vi "Joystick interpolation Full.vi"(8 "array":dbl[](array[numeric]), 9 "Numeric":dbl=1000.0 format="%#_13g", 10 "Joystick Sim":dbl(slide) scale=-1.0..1.0, 11 "method":i32(ring)=3 items=["nearest", "linear", "spline", "cubic Hermite", "Lagrange"]) -> (3 "Power":dbl(slide) scale=-1.0..1.0)   [LabVIEW 2017]
uses:
  <vilib>/Analysis/1siggen.llb/Ramp Pattern by Delta.vi
  <vilib>/gmath/NI_Gmath.lvlib
  <vilib>/Analysis/NI_AALBase.lvlib
panel:
  out "Interpolated Data":dbl[][](array[numeric])
  out "1D Interpolation Graph":cluster{"yi":dbl[], "ramp data":dbl[]}[](graph)
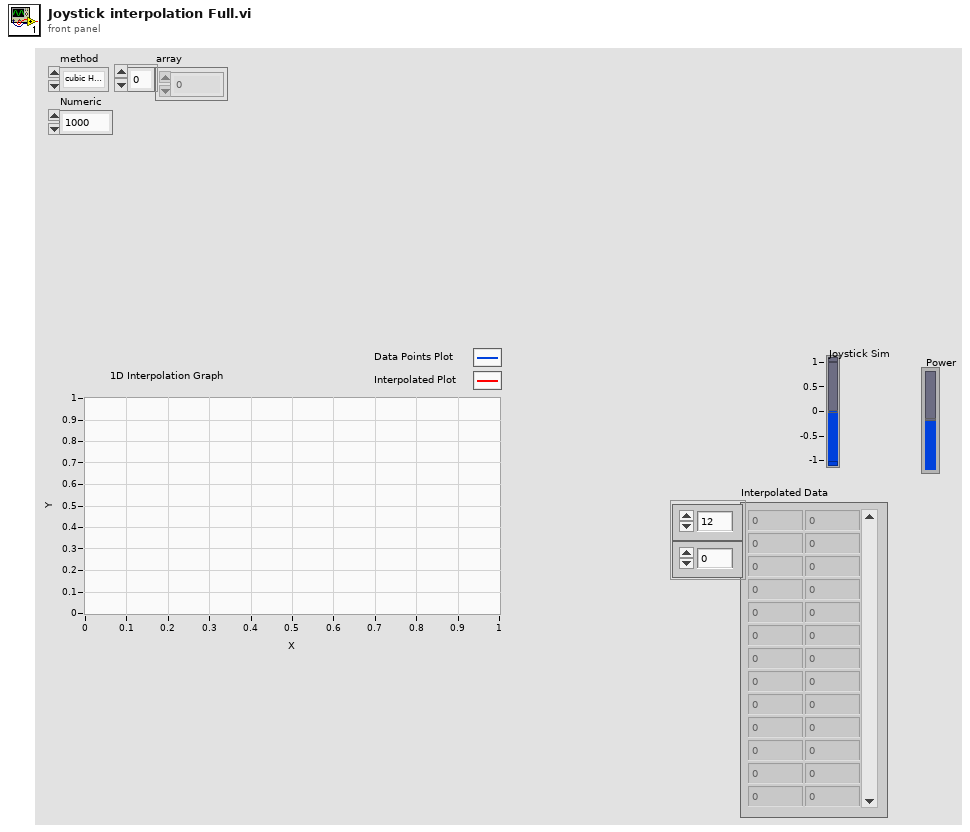
[diagram p1: front panel]
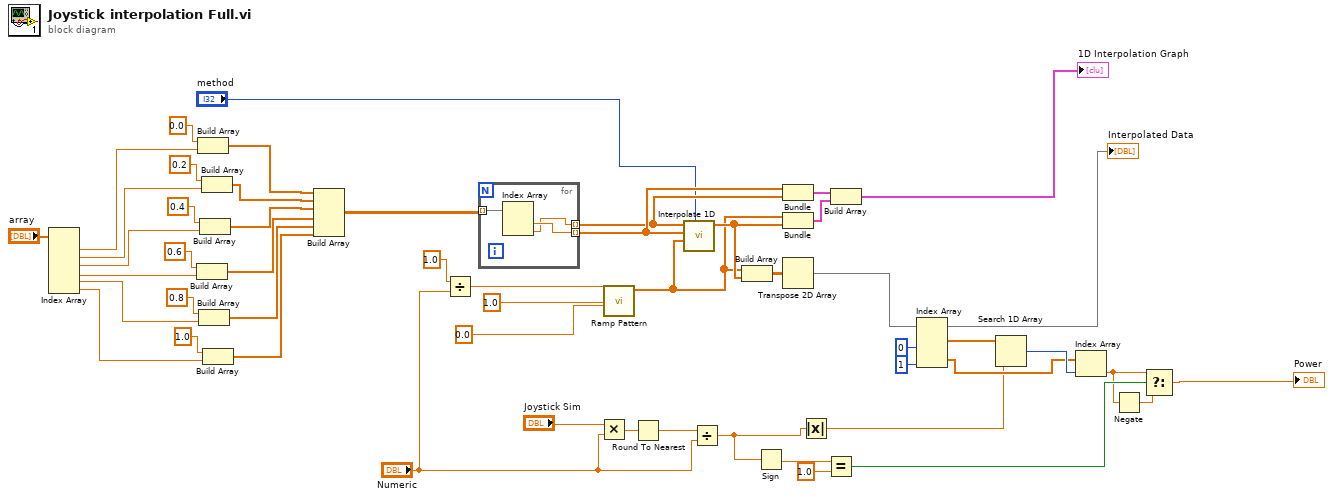
[diagram p0: block diagram]
diagram:
  n1 = Index Array(array="array") -> (element #1=w7:dbl, element #2=w5:dbl, element #3=w4:dbl, element #4=w3:dbl, element #5=w2:dbl, element #6=w1:dbl)  [unwired: 6 in]
  n2 = Build Array(0.6 ("element"), w3) -> (w44:dbl[])
  n3 = Build Array(0.0 ("element"), w7) -> (w47:dbl[])
  n4 = Build Array(0.8 ("element"), w2) -> (w36:dbl[])
  n5 = Build Array(0.4 ("element"), w4) -> (w45:dbl[])
  n6 = Build Array(0.2 ("element"), w5) -> (w46:dbl[])
  n7 = Build Array(1.0 ("element"), w1) -> (w35:dbl[])
  n8 = Build Array(w47, w46, w45, w44, w36, w35) -> (w13:dbl[][])
  n9 = Divide(x=1.0 ("delta"), y="Numeric") -> (x/y=w8:dbl)
  n10 = for {
    tunnel: [w52] -> w20 mode=indexing
    tunnel: [w53] -> w21 mode=indexing
    tunnel: w13 -> [w54] mode=indexing
    n11 = Index Array(array=w54) -> (element #1=w53:dbl, element #2=w52:dbl)  [unwired: 2 in]
  }
  n12 = Multiply(x="Joystick Sim", y="Numeric") -> (x*y=w33:dbl)
  n13 = call-poly <vilib>:"Ramp Pattern.vi"("start"=0.0, "end"=1.0, "delta"=w8) -> ("Ramp Pattern"=w17:dbl[])  [unwired: 6 in, 2 out]
  n14 = Round To Nearest(number=w33) -> (nearest integer value=w32:dbl)
  n15 = call <vilib>:"Interpolate 1D.vi"("method"="method", "xi"=w17, "X"=w21, "Y"=w20) -> ("yi"=w18:dbl[])  [unwired: 5 in, 2 out]
  n16 = Divide(x=w32, y="Numeric") -> (x/y=w31:dbl)
  n17 = Build Array(w17, w18) -> (w19:dbl[][])
  n18 = Sign(1:w31) -> (0:w29:dbl)
  n19 = Bundle(w21, w20) -> (w22:cluster{dbl[], dbl[]})  [unwired: 1 in]
  n20 = Bundle("Ramp Pattern"=w17, "yi"=w18) -> (w23:cluster{"Ramp Pattern":dbl[], "yi":dbl[]})  [unwired: 1 in]
  n21 = Transpose 2D Array(2D array=w19) -> (transposed array=w11:dbl[][])
  "Interpolated Data" <- w11
  n22 = Absolute Value(x=w31) -> (abs(x)=w30:dbl)
  n23 = Equal?(x=w29, y=1.0) -> (x = y?=w27:bool)
  n24 = Build Array(w22, w23) -> (→"1D Interpolation Graph":cluster{"Ramp Pattern":dbl[], "yi":dbl[]}[])
  n25 = Index Array(array=w11, index (col) #1=0 ("disabled index (col)"), index (col) #2=1 ("index (col)")) -> (element #1=w39:dbl[], element #2=w40:dbl[])  [unwired: 2 in]
  n26 = Search 1D Array(1D array=w39, element=w30) -> (index of element=w43:i32)  [unwired: 1 in]
  n27 = Index Array(array=w40, index=w43) -> (element=w25:dbl)
  n28 = Negate(x=w25) -> (-x=w26:dbl)
  n29 = Select(t=w25, s=w27, f=w26) -> (s? t:f=→"Power":dbl)
